vi "Flow FGV.vi"(7 "Write":bool, 8 "error in (no error)":errorcluster, 11 "Flow In (ml/min)":dbl) -> (0 "error out":errorcluster, 3 "Flow Out (ml/min)":dbl)   [LabVIEW 2021]
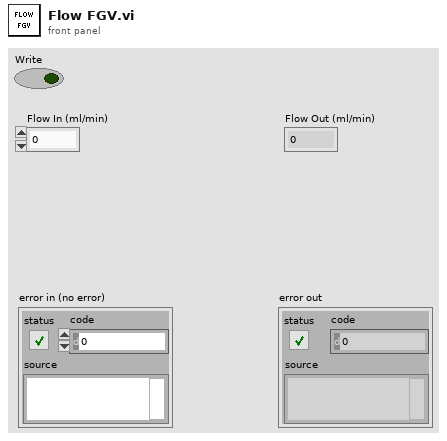
[diagram p1: front panel]
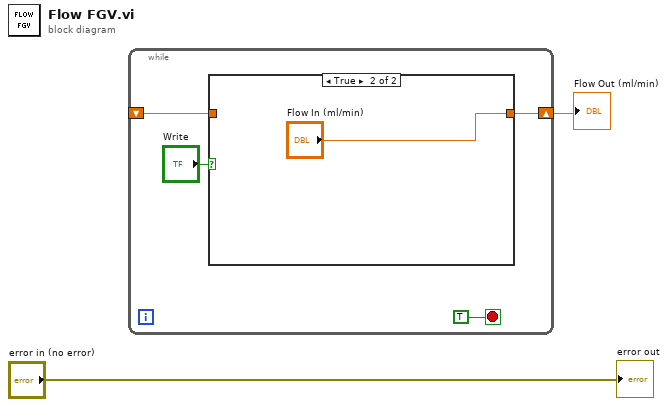
[diagram p0: block diagram]
diagram:
  n1 = while {
    shift-right: [w4] -> w2
    shift-left: _ -> [w3]
    stop <- TRUE stop-if-true
    n2 = case shown="True" "Write" {
      tunnel: [w7 "Flow In (ml/min)"] -> w4
      tunnel: w3 -> [w7 _]
      frame False {
      }
      frame True {
      }
    }
  }
  "Flow Out (ml/min)" <- w2
  "error out" <- "error in (no error)"
